vi "ChangeConfigGUI.vi"(4 "error in (no error)":errorcluster, 5 "Configuration Flags":T3, 6 "Configuration Read":T4 {"Select Mode:" items=["Custom", "Imaging", "300 All", "600 UV", "600 Blue", "600 Mid", "600 Red", "1200 m0", "1200 m1", "1200 m2", "1200 m3", "1200 m4", "1200 m5", "1200 m6", "1200 m7", "1200 RESOLVE", "400 m1", "400 m2", "930 m1", "930 m2", "930 m3", "930 m4", "930 m5", "930 m6", "400KL"]}, 7 "Cam Focus":dbl) -> (0 "error out":errorcluster, 1 "Script":T1[](array[typedef]), 2 "Targets":T2 {"Select Mode:" items=["Custom", "Imaging", "300 All", "600 UV", "600 Blue", "600 Mid", "600 Red", "1200 m0", "1200 m1", "1200 m2", "1200 m3", "1200 m4", "1200 m5", "1200 m6", "1200 m7", "1200 RESOLVE", "400 m1", "400 m2", "930 m1", "930 m2", "930 m3", "930 m4", "930 m5", "930 m6", "400KL"]})   [LabVIEW 2015]
doc: "This GUI interprets supplied configuration information and displays it to the user. It compares the target configuration to the machine state (what components are loaded) and checks for compatibility. If the user choses to start a move, an enumerated script is output that can be used to start a sequence of moves."
uses:
  GSCS Scripting/Utils/GSP_ObsConfig.llb/configuration.ctl
  GSCS Scripting/Utils/Script_actions.ctl
  Dialog/dialog_messages.ctl
  GSP_GUI_global.vi
panel:
  in  "Something not loaded?":bool
  out "Date":string
  out "User":string
  out "Name":string
  in  "Configuration":i32(listbox)
  # "Systems will finish any current scripts \nbefore beginning the configuration\nchange."
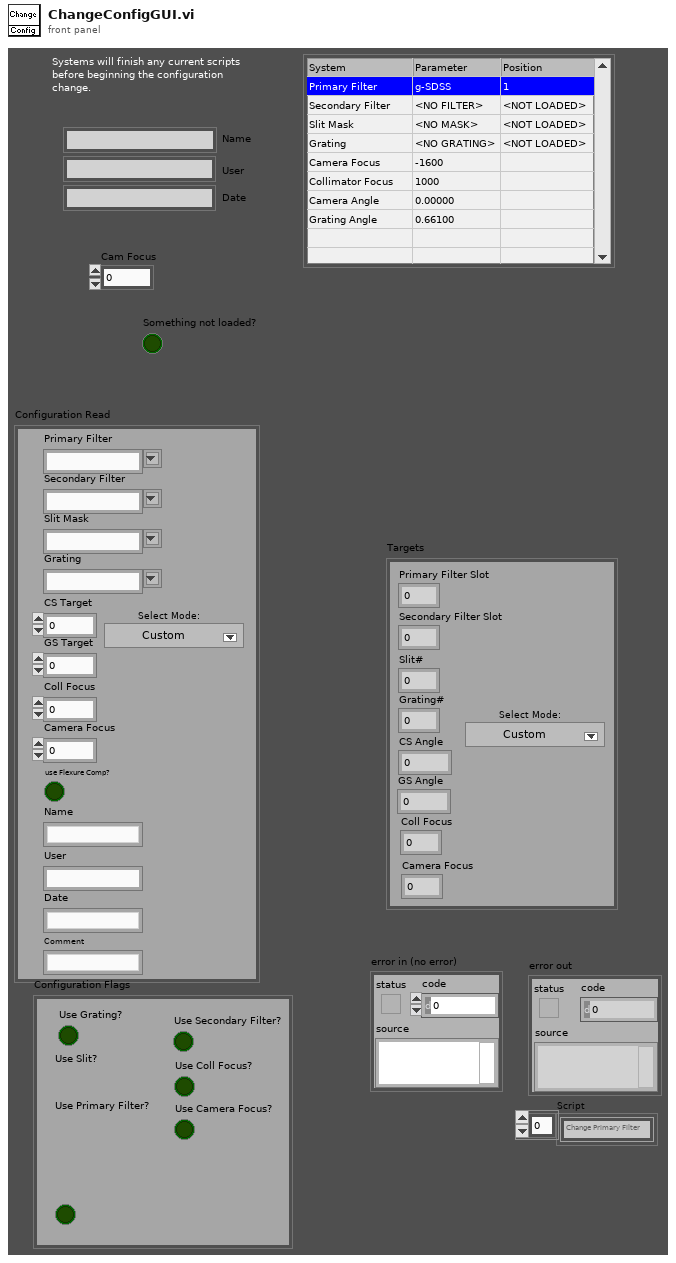
[diagram p1: front panel]
types:
  T1 = typedef "Script_actions.ctl" = enum16{"Change Primary Filter", "Change Secondary Filter", "Change Collimator Focus", "Change Camera Focus", "Change Grating", "Change Angles", "Change Slit Mask", "Change WAVMODE"}
  T2 = cluster{"Primary Filter Slot":i32, "Secondary Filter Slot":i32, "Slit#":i32, "Grating#":i32, "CS Angle":dbl, "GS Angle":dbl, "Coll Focus":i32, "Camera Focus":i32, "Select Mode:":u16}
  T3 = cluster{"Use Grating?":bool, "Use Slit?":bool, "Use Primary Filter?":bool, "Use Secondary Filter?":bool, "Use Coll Focus?":bool, "Use Camera Focus?":bool}
  T4 = typedef "configuration.ctl" = cluster{"Primary Filter":string, "Secondary Filter":string, "Slit Mask":string, "Grating":string, "CS Target":dbl, "GS Target":dbl, "Coll Focus":i32, "Camera Focus":i32, "Name":string, "User":string, "Date":string, "Comment":string, "use Flexure Comp?":bool, "Select Mode:":u16}
  T5 = cluster{"Primary Filter Slot":i32, "Secondary Filter Slot":i32, "Slit#":i32, "Grating#":i32, "CS Angle":dbl, "GS Angle":dbl, "Coll Focus":i32, "Camera Focus":i32, "Select Mode":i32}
  T6 = typedef "dialog_messages.ctl" = enum16{"Custom", "Incompatible Config"}
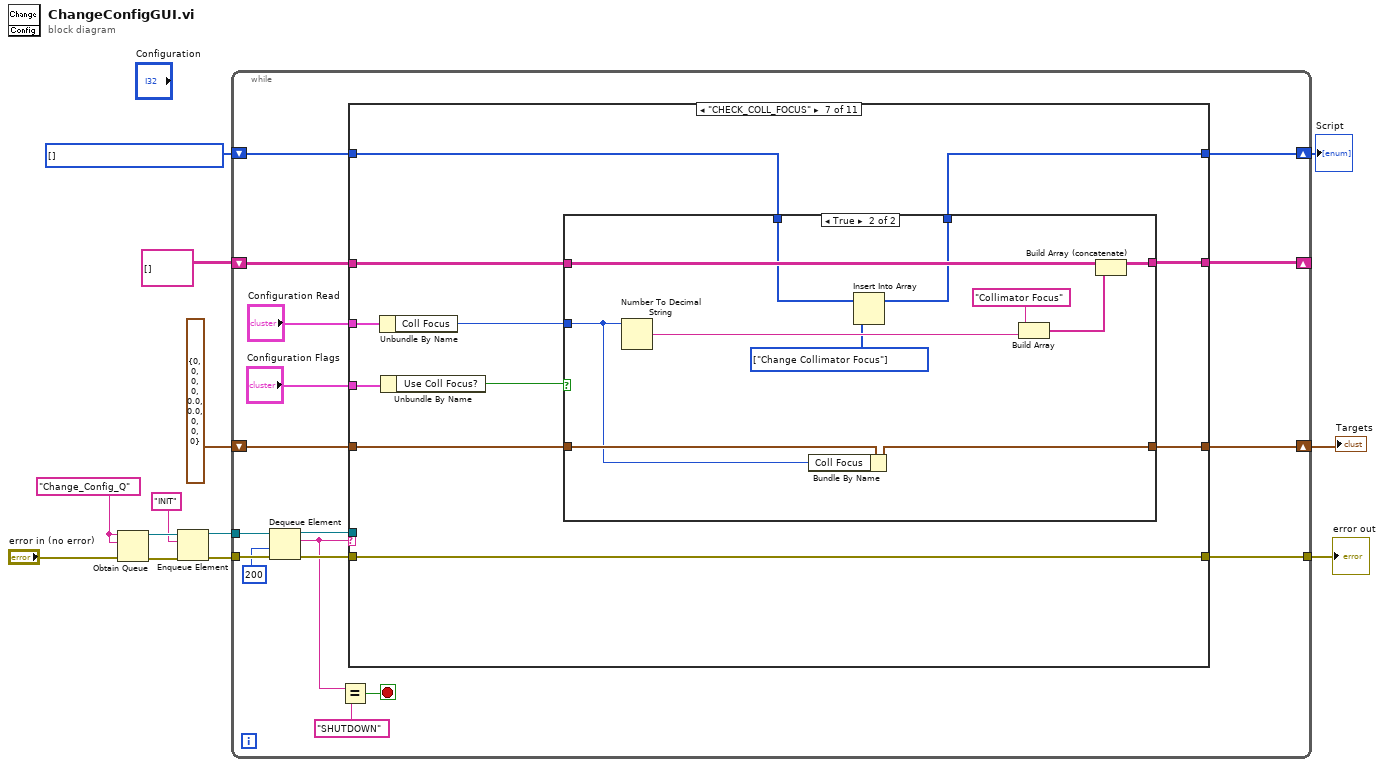
[diagram p0: block diagram]
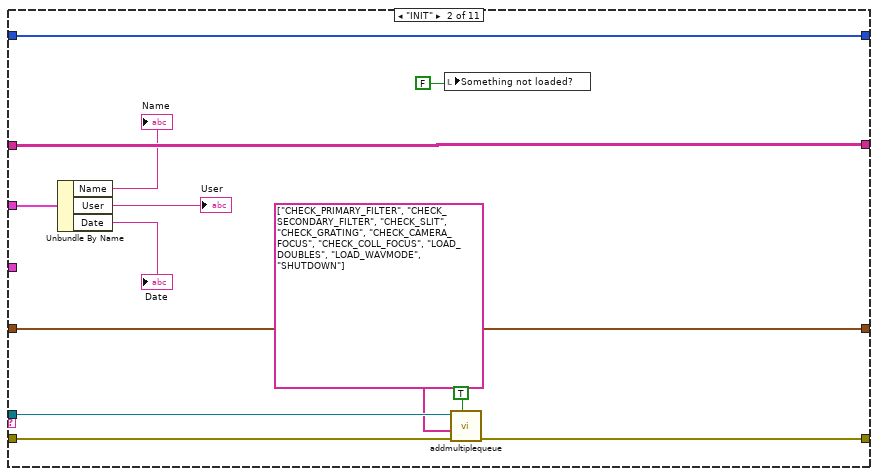
[diagram p3: hidden frame]
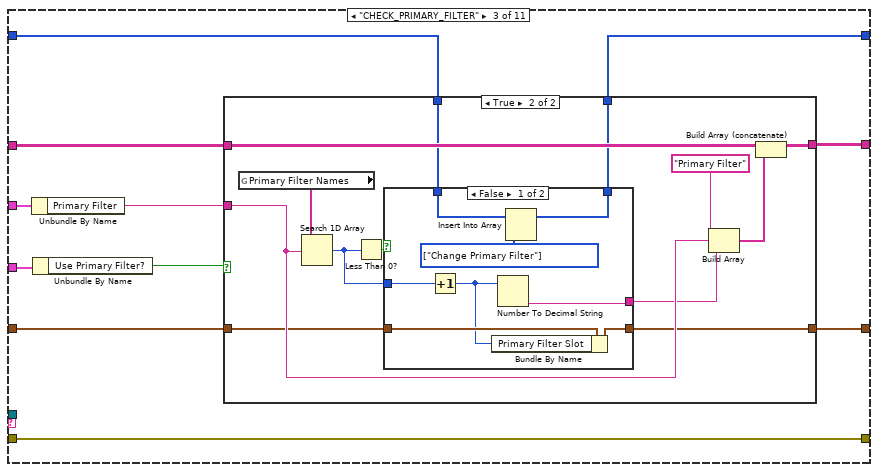
[diagram p4: hidden frame]
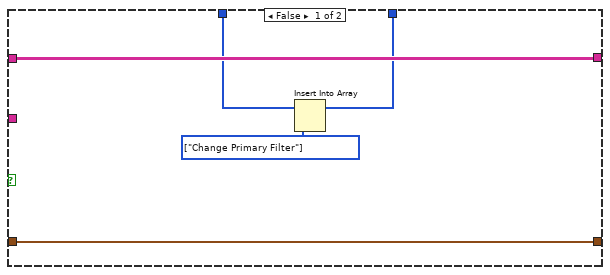
[diagram p5: hidden frame]
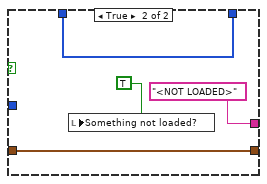
[diagram p6: hidden frame]
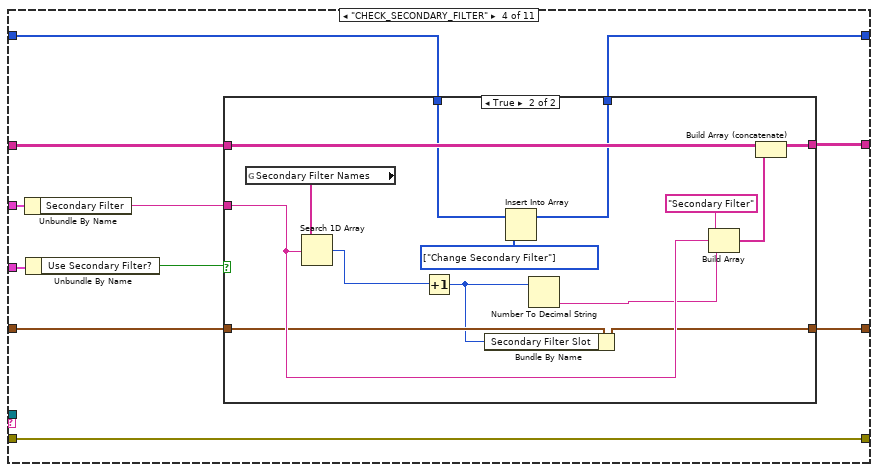
[diagram p7: hidden frame]
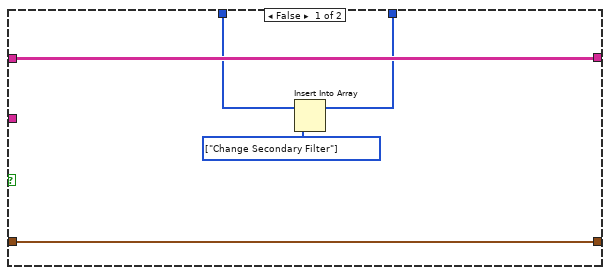
[diagram p8: hidden frame]
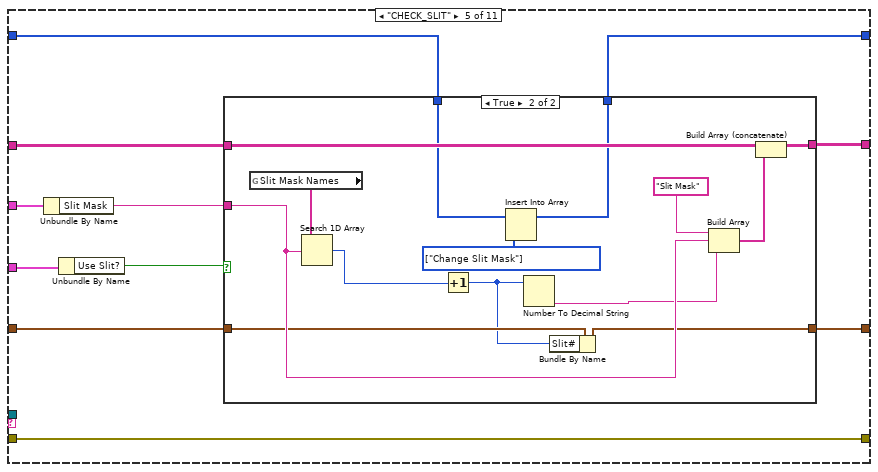
[diagram p9: hidden frame]
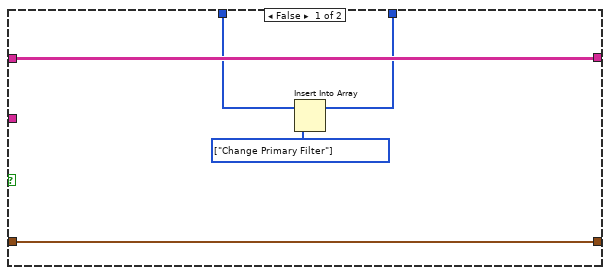
[diagram p10: hidden frame]
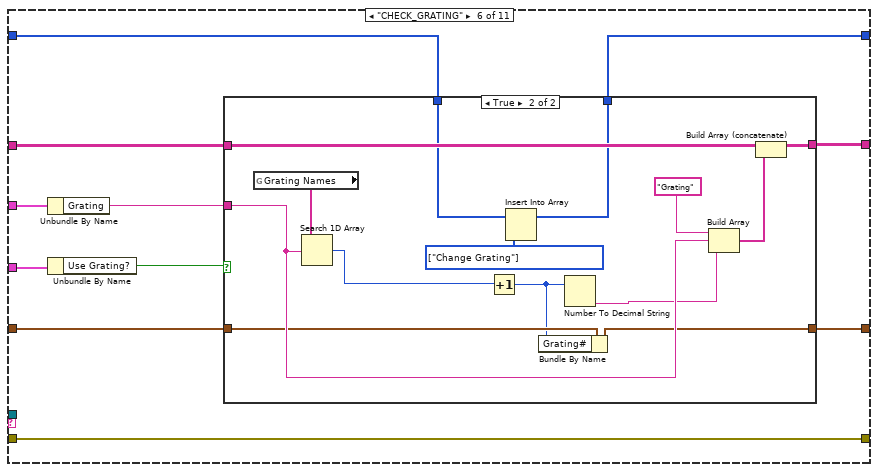
[diagram p11: hidden frame]
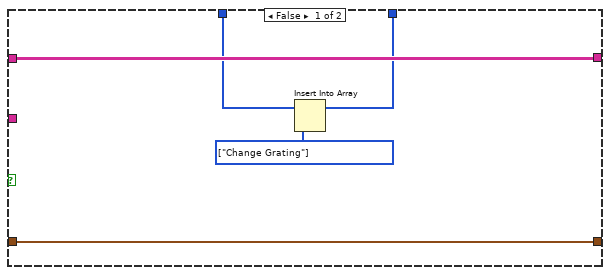
[diagram p12: hidden frame]
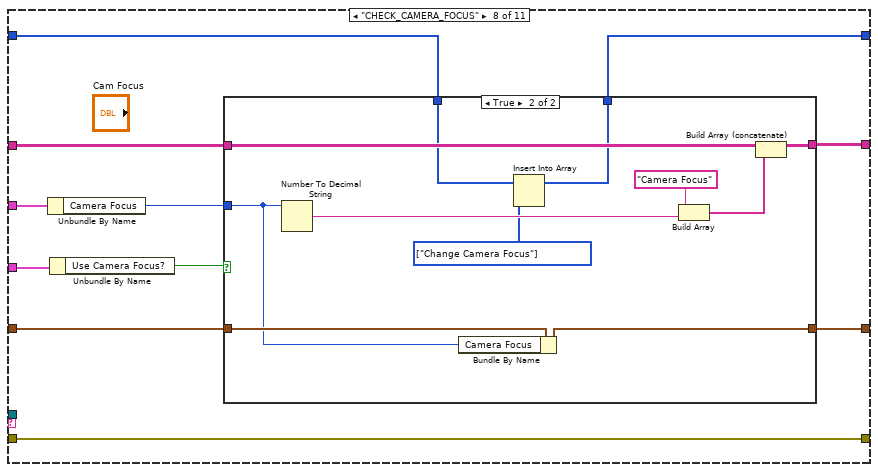
[diagram p14: hidden frame]
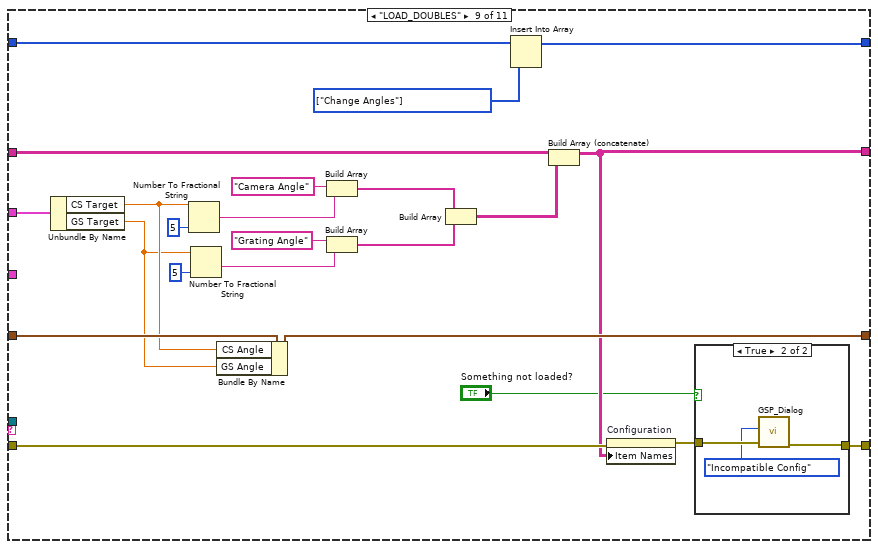
[diagram p16: hidden frame]
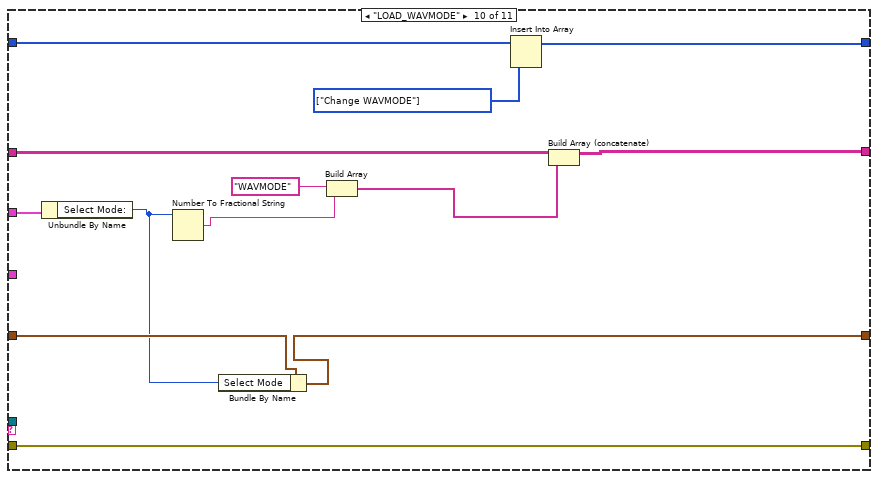
[diagram p18: hidden frame]
diagram:
  w4 = T1[] [] items=["Change Primary Filter", "Change Secondary Filter", "Change Collimator Focus", "Change Camera Focus", "Change Grating", "Change Angles", "Change Slit Mask", "Change WAVMODE"]
  w11 = "Change_Config_Q" ("name (unnamed)")
  n1 = Obtain Queue(name (unnamed)=w11, element data type=w11, error in (no error)="error in (no error)") -> (queue out=w8:refnum<queue>, error out=w9:errorcluster)  [unwired: 2 in, 1 out]
  n2 = Enqueue Element(queue=w8, element="INIT", error in (no error)=w9) -> (queue out=w7:refnum<queue>, error out=w10:errorcluster)  [unwired: 1 in, 1 out]
  n3 = while {
    tunnel: w10 -> [w29]
    tunnel: [w30] -> w13
    tunnel: w7 -> [w27]
    shift-right: [w20] -> _
    shift-left: string[][] [] -> [w21]
    shift-right: [w16] -> w1
    shift-left: w4 -> [w17]
    shift-right: [w14] -> w2
    shift-left: T5 {"Primary Filter Slot"=0, "Secondary Filter Slot"=0, "Slit#"=0, "Grating#"=0, "CS Angle"=0.0, "GS Angle"=0.0, "Coll Focus"=0, "Camera Focus"=0, "Select Mode"=0} ("Targets") -> [w15]
    stop <- w23 stop-if-true
    n4 = Dequeue Element(queue=w27, timeout in ms (-1)=200, error in (no error)=w29) -> (queue out=w26:refnum<queue>, element=w25:string, error out=w28:errorcluster)  [unwired: 1 out]
    n5 = Equal?(x=w25, y="SHUTDOWN") -> (x = y?=w23:bool)
    n6 = case shown="\"CHECK_COLL_FOCUS\"" w25 {
      tunnel: w28 -> [w31 w42 w52 w93 w123 w153 w183 w209 w236 w262 w272]
      tunnel: [w31 w40 w52 w93 w123 w153 w183 w209 w230 w262 w272] -> w30
      tunnel: w26 -> [_ w41 _ _ _ _ _ _ _ _ _]
      tunnel: w21 -> [w34 w47 w56 w97 w127 w157 w187 w212 w251 w268 w271]
      tunnel: [w34 w47 w53 w94 w124 w154 w184 w210 w235 w266 w271] -> w20
      tunnel: "Configuration Read" -> [_ w46 w58 w99 w129 w159 w189 w214 w241 w260 _]
      tunnel: "Configuration Flags" -> [_ _ w57 w98 w128 w158 w188 w213 _ _ _]
      tunnel: w17 -> [w33 w38 w51 w92 w122 w152 w182 w208 w234 w265 w269]
      tunnel: [w33 w38 w50 w91 w121 w151 w181 w207 w233 w264 w269] -> w16
      tunnel: w15 -> [w32 w37 w49 w90 w120 w150 w180 w206 w240 w259 w270]
      tunnel: [w32 w37 w48 w89 w119 w149 w179 w205 w239 w258 w270] -> w14
      frame "", Default {
      }
      frame "INIT" {
        n7 = Unbundle By Name(w46) -> ("Name"=→"Name":string, "User"=→"User":string, "Date"=→"Date":string)
        n8 = local write "Something not loaded?"(FALSE) -> ()
        n9 = call "addmultiplequeue.vi"("Add All (false)"=TRUE, "error in (no error)"=w42, "Strings to Add"=string[] ["CHECK_PRIMARY_FILTER", "CHECK_SECONDARY_FILTER", "CHECK_SLIT", "CHECK_GRATING", "CHECK_CAMERA_FOCUS", "CHECK_COLL_FOCUS", "LOAD_DOUBLES", "LOAD_WAVMODE", "SHUTDOWN"], "queue"=w41) -> ("error out"=w40:errorcluster)  [unwired: 3 in, 1 out]
      }
      frame "CHECK_PRIMARY_FILTER" {
        n10 = Unbundle By Name(w58) -> ("Primary Filter"=w54:string)
        n11 = Unbundle By Name(w57) -> ("Use Primary Filter?"=w55:bool)
        n12 = case shown="True" w55 {
          tunnel: w56 -> [w63 w72]
          tunnel: w54 -> [_ w70]
          tunnel: [w63 w73] -> w53
          tunnel: w51 -> [w62 w67]
          tunnel: [w61 w66] -> w50
          tunnel: w49 -> [w60 w65]
          tunnel: [w60 w64] -> w48
          frame False {
            w59 = T1[] [enum."Change Primary Filter"] items=["Change Primary Filter", "Change Secondary Filter", "Change Collimator Focus", "Change Camera Focus", "Change Grating", "Change Angles", "Change Slit Mask", "Change WAVMODE"]
            n13 = Insert Into Array(array=w62, new element=w59) -> (w61:T1[])  [unwired: 1 in]
          }
          frame True {
            n14 = global read "GSP_GUI_global.vi" "Primary Filter Names"() -> (w76:string[])
            n15 = Search 1D Array(1D array=w76, element=w70) -> (index of element=w74:i32)  [unwired: 1 in]
            n16 = Less Than 0?(x=w74) -> (x < 0?=w75:bool)
            n17 = case shown="False" w75 {
              tunnel: w74 -> [w79 _]
              tunnel: [w84 "<NOT LOADED>"] -> w69
              tunnel: w67 -> [w83 w87]
              tunnel: [w82 w87] -> w66
              tunnel: w65 -> [w81 w86]
              tunnel: [w80 w86] -> w64
              frame False {
                w77 = T1[] [enum."Change Primary Filter"] items=["Change Primary Filter", "Change Secondary Filter", "Change Collimator Focus", "Change Camera Focus", "Change Grating", "Change Angles", "Change Slit Mask", "Change WAVMODE"]
                n18 = Increment(x=w79) -> (x+1=w78:i32)
                n19 = Bundle By Name(cluster=w81, "Primary Filter Slot"=w78) -> (w80:T5)
                n20 = Number To Decimal String(number=w78) -> (decimal integer string=w84:string)  [unwired: 1 in]
                n21 = Insert Into Array(array=w83, new element=w77) -> (w82:T1[])  [unwired: 1 in]
              }
              frame True {
                n22 = local write "Something not loaded?"(TRUE) -> ()
              }
            }
            n23 = Build Array("Primary Filter", w70, w69) -> (w68:string[])
            n24 = Build Array (concatenate)(w72, w68) -> (w73:string[][])
          }
        }
      }
      frame "CHECK_SECONDARY_FILTER" {
        n25 = Unbundle By Name(w99) -> ("Secondary Filter"=w95:string)
        n26 = Unbundle By Name(w98) -> ("Use Secondary Filter?"=w96:bool)
        n27 = case shown="True" w96 {
          tunnel: w97 -> [w104 w115]
          tunnel: w95 -> [_ w113]
          tunnel: [w104 w116] -> w94
          tunnel: w92 -> [w103 w110]
          tunnel: [w102 w109] -> w91
          tunnel: w90 -> [w101 w108]
          tunnel: [w101 w107] -> w89
          frame False {
            w100 = T1[] [enum."Change Secondary Filter"] items=["Change Primary Filter", "Change Secondary Filter", "Change Collimator Focus", "Change Camera Focus", "Change Grating", "Change Angles", "Change Slit Mask", "Change WAVMODE"]
            n28 = Insert Into Array(array=w103, new element=w100) -> (w102:T1[])  [unwired: 1 in]
          }
          frame True {
            w105 = T1[] [enum."Change Secondary Filter"] items=["Change Primary Filter", "Change Secondary Filter", "Change Collimator Focus", "Change Camera Focus", "Change Grating", "Change Angles", "Change Slit Mask", "Change WAVMODE"]
            n29 = global read "GSP_GUI_global.vi" "Secondary Filter Names"() -> (w118:string[])
            n30 = Search 1D Array(1D array=w118, element=w113) -> (index of element=w117:i32)  [unwired: 1 in]
            n31 = Increment(x=w117) -> (x+1=w106:i32)
            n32 = Bundle By Name(cluster=w108, "Secondary Filter Slot"=w106) -> (w107:T5)
            n33 = Insert Into Array(array=w110, new element=w105) -> (w109:T1[])  [unwired: 1 in]
            n34 = Number To Decimal String(number=w106) -> (decimal integer string=w112:string)  [unwired: 1 in]
            n35 = Build Array("Secondary Filter", w113, w112) -> (w111:string[])
            n36 = Build Array (concatenate)(w115, w111) -> (w116:string[][])
          }
        }
      }
      frame "CHECK_SLIT" {
        n37 = Unbundle By Name(w129) -> ("Slit Mask"=w125:string)
        n38 = Unbundle By Name(w128) -> ("Use Slit?"=w126:bool)
        n39 = case shown="True" w126 {
          tunnel: w127 -> [w134 w145]
          tunnel: w125 -> [_ w143]
          tunnel: [w134 w146] -> w124
          tunnel: w122 -> [w133 w140]
          tunnel: [w132 w139] -> w121
          tunnel: w120 -> [w131 w138]
          tunnel: [w131 w137] -> w119
          frame False {
            w130 = T1[] [enum."Change Primary Filter"] items=["Change Primary Filter", "Change Secondary Filter", "Change Collimator Focus", "Change Camera Focus", "Change Grating", "Change Angles", "Change Slit Mask", "Change WAVMODE"]
            n40 = Insert Into Array(array=w133, new element=w130) -> (w132:T1[])  [unwired: 1 in]
          }
          frame True {
            w135 = T1[] [enum."Change Slit Mask"] items=["Change Primary Filter", "Change Secondary Filter", "Change Collimator Focus", "Change Camera Focus", "Change Grating", "Change Angles", "Change Slit Mask", "Change WAVMODE"]
            n41 = global read "GSP_GUI_global.vi" "Slit Mask Names"() -> (w148:string[])
            n42 = Search 1D Array(1D array=w148, element=w143) -> (index of element=w147:i32)  [unwired: 1 in]
            n43 = Increment(x=w147) -> (x+1=w136:i32)
            n44 = Insert Into Array(array=w140, new element=w135) -> (w139:T1[])  [unwired: 1 in]
            n45 = Number To Decimal String(number=w136) -> (decimal integer string=w142:string)  [unwired: 1 in]
            n46 = Bundle By Name(cluster=w138, "Slit#"=w136) -> (w137:T5)
            n47 = Build Array("Slit Mask", w143, w142) -> (w141:string[])
            n48 = Build Array (concatenate)(w145, w141) -> (w146:string[][])
          }
        }
      }
      frame "CHECK_GRATING" {
        n49 = Unbundle By Name(w159) -> ("Grating"=w155:string)
        n50 = Unbundle By Name(w158) -> ("Use Grating?"=w156:bool)
        n51 = case shown="True" w156 {
          tunnel: w157 -> [w164 w175]
          tunnel: w155 -> [_ w173]
          tunnel: [w164 w176] -> w154
          tunnel: w152 -> [w163 w170]
          tunnel: [w162 w169] -> w151
          tunnel: w150 -> [w161 w168]
          tunnel: [w161 w167] -> w149
          frame False {
            w160 = T1[] [enum."Change Grating"] items=["Change Primary Filter", "Change Secondary Filter", "Change Collimator Focus", "Change Camera Focus", "Change Grating", "Change Angles", "Change Slit Mask", "Change WAVMODE"]
            n52 = Insert Into Array(array=w163, new element=w160) -> (w162:T1[])  [unwired: 1 in]
          }
          frame True {
            w165 = T1[] [enum."Change Grating"] items=["Change Primary Filter", "Change Secondary Filter", "Change Collimator Focus", "Change Camera Focus", "Change Grating", "Change Angles", "Change Slit Mask", "Change WAVMODE"]
            n53 = global read "GSP_GUI_global.vi" "Grating Names"() -> (w178:string[])
            n54 = Search 1D Array(1D array=w178, element=w173) -> (index of element=w177:i32)  [unwired: 1 in]
            n55 = Increment(x=w177) -> (x+1=w166:i32)
            n56 = Insert Into Array(array=w170, new element=w165) -> (w169:T1[])  [unwired: 1 in]
            n57 = Bundle By Name(cluster=w168, "Grating#"=w166) -> (w167:T5)
            n58 = Number To Decimal String(number=w166) -> (decimal integer string=w172:string)  [unwired: 1 in]
            n59 = Build Array("Grating", w173, w172) -> (w171:string[])
            n60 = Build Array (concatenate)(w175, w171) -> (w176:string[][])
          }
        }
      }
      frame "CHECK_COLL_FOCUS" {
        n61 = Unbundle By Name(w189) -> ("Coll Focus"=w185:i32)
        n62 = Unbundle By Name(w188) -> ("Use Coll Focus?"=w186:bool)
        n63 = case shown="True" w186 {
          tunnel: w187 -> [w192 w202]
          tunnel: w185 -> [_ w195]
          tunnel: [w192 w203] -> w184
          tunnel: w182 -> [w190 w199]
          tunnel: [w190 w198] -> w181
          tunnel: w180 -> [w191 w196]
          tunnel: [w191 w194] -> w179
          frame False {
          }
          frame True {
            w193 = T1[] [enum."Change Collimator Focus"] items=["Change Primary Filter", "Change Secondary Filter", "Change Collimator Focus", "Change Camera Focus", "Change Grating", "Change Angles", "Change Slit Mask", "Change WAVMODE"]
            n64 = Number To Decimal String(number=w195) -> (decimal integer string=w197:string)  [unwired: 1 in]
            n65 = Bundle By Name(cluster=w196, "Coll Focus"=w195) -> (w194:T5)
            n66 = Insert Into Array(array=w199, new element=w193) -> (w198:T1[])  [unwired: 1 in]
            n67 = Build Array("Collimator Focus", w197) -> (w200:string[])
            n68 = Build Array (concatenate)(w202, w200) -> (w203:string[][])
          }
        }
      }
      frame "CHECK_CAMERA_FOCUS" {
        n69 = Unbundle By Name(w214) -> ("Camera Focus"=w204:i32)
        n70 = Unbundle By Name(w213) -> ("Use Camera Focus?"=w211:bool)
        n71 = case shown="True" w211 {
          tunnel: w212 -> [w217 w227]
          tunnel: w204 -> [_ w220]
          tunnel: [w217 w228] -> w210
          tunnel: w208 -> [w215 w224]
          tunnel: [w215 w223] -> w207
          tunnel: w206 -> [w216 w221]
          tunnel: [w216 w219] -> w205
          frame False {
          }
          frame True {
            w218 = T1[] [enum."Change Camera Focus"] items=["Change Primary Filter", "Change Secondary Filter", "Change Collimator Focus", "Change Camera Focus", "Change Grating", "Change Angles", "Change Slit Mask", "Change WAVMODE"]
            n72 = Number To Decimal String(number=w220) -> (decimal integer string=w222:string)  [unwired: 1 in]
            n73 = Bundle By Name(cluster=w221, "Camera Focus"=w220) -> (w219:T5)
            n74 = Insert Into Array(array=w224, new element=w218) -> (w223:T1[])  [unwired: 1 in]
            n75 = Build Array("Camera Focus", w222) -> (w225:string[])
            n76 = Build Array (concatenate)(w227, w225) -> (w228:string[][])
          }
        }
      }
      frame "LOAD_DOUBLES" {
        w229 = T1[] [enum."Change Angles"] items=["Change Primary Filter", "Change Secondary Filter", "Change Collimator Focus", "Change Camera Focus", "Change Grating", "Change Angles", "Change Slit Mask", "Change WAVMODE"]
        n77 = Unbundle By Name(w241) -> ("CS Target"=w238:dbl, "GS Target"=w237:dbl)
        n78 = Number To Fractional String(number=w238, precision (6)=i16 5) -> (F-format string=w247:string)  [unwired: 2 in]
        n79 = Number To Fractional String(number=w237, precision (6)=i16 5) -> (F-format string=w245:string)  [unwired: 2 in]
        n80 = Bundle By Name(cluster=w240, "CS Angle"=w238, "GS Angle"=w237) -> (w239:T5)
        n81 = Build Array("Camera Angle", w247) -> (w244:string[])
        n82 = Build Array("Grating Angle", w245) -> (w243:string[])
        n83 = Build Array(w244, w243) -> (w242:string[][])
        n84 = Insert Into Array(array=w234, new element=w229) -> (w233:T1[])  [unwired: 1 in]
        n85 = Build Array (concatenate)(w251, w242) -> (w235:string[][])
        n86 = property on="Configuration" class="MCListbox (strict)"(error in=w236, "Item Names"=w235) -> (error out=w231:errorcluster)  [unwired: 1 in, 1 out]
        n87 = case shown="True" "Something not loaded?" {
          tunnel: w231 -> [w252 w255]
          tunnel: [w252 w253] -> w230
          frame False {
          }
          frame True {
            n88 = call "GSP_Dialog.vi"("error in (no error)"=w255, "Messages"=dialog_messages."Incompatible Config") -> ("error out"=w253:errorcluster)  [unwired: 5 in]
          }
        }
      }
      frame "LOAD_WAVMODE" {
        w263 = T1[] [enum."Change WAVMODE"] items=["Change Primary Filter", "Change Secondary Filter", "Change Collimator Focus", "Change Camera Focus", "Change Grating", "Change Angles", "Change Slit Mask", "Change WAVMODE"]
        n89 = Unbundle By Name(w260) -> ("Select Mode:"=w256:u16)
        n90 = Number To Fractional String(number=w256) -> (F-format string=w257:string)  [unwired: 3 in]
        n91 = Bundle By Name(cluster=w259, "Select Mode"=w256) -> (w258:T5)
        n92 = Build Array("WAVMODE", w257) -> (w261:string[])
        n93 = Insert Into Array(array=w265, new element=w263) -> (w264:T1[])  [unwired: 1 in]
        n94 = Build Array (concatenate)(w268, w261) -> (w266:string[][])
      }
      frame "SHUTDOWN" {
      }
    }
  }
  "error out" <- w13
  "Targets" <- w2
  "Script" <- w1
